vi "Get Test Limits Source File Name.vi"(8 "error in (no error)":errorcluster, 11 "Path":path) -> (0 "error out":errorcluster, 3 "Source File":string)   [LabVIEW 2025, in "File System.lvlib"]
uses:
  File System.lvlib
  <vilib>/Utility/file.llb/Read Delimited Spreadsheet (string).vi
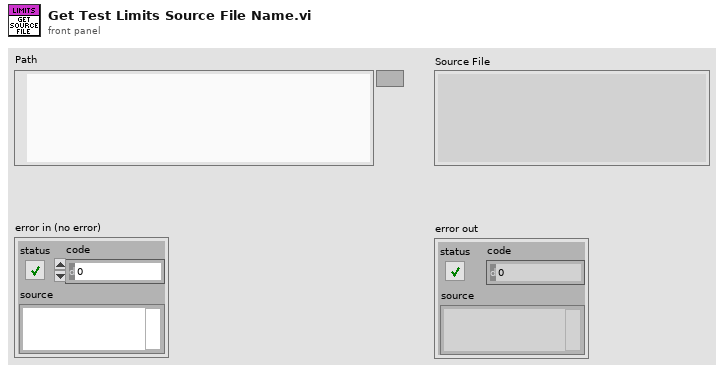
[diagram p1: front panel]
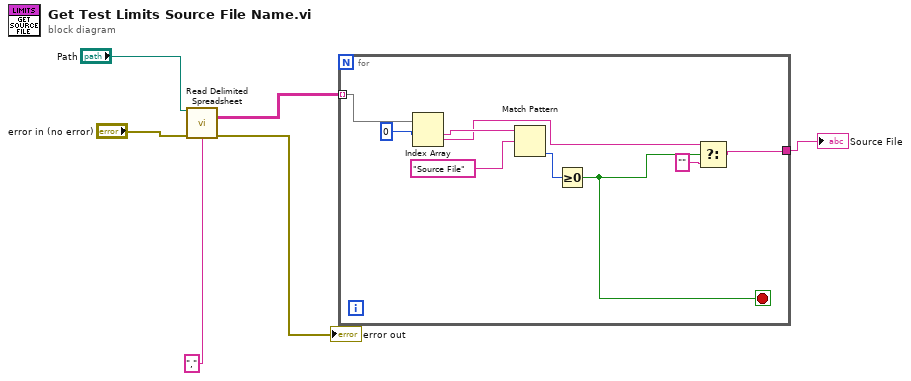
[diagram p0: block diagram]
diagram:
  n1 = call-poly <vilib>:"Read Delimited Spreadsheet.vi"("file path (dialog if empty)"="Path", "error in (no error)"="error in (no error)", "delimiter (\\t)"="," ("delimiter (\\t)")) -> ("all rows"=w2:string[][], "error out"=→"error out":errorcluster)  [unwired: 7 in, 4 out]
  n2 = for {
    tunnel: w2 -> [w15] mode=indexing
    tunnel: [w7] -> w1
    stop <- w10 stop-if-true
    n3 = Index Array(array=w15, index #1=0 ("index")) -> (element #1=w13:string, element #2=w9:string)  [unwired: 1 in]
    n4 = Match Pattern(string=w13, regular expression="Source File") -> (offset past match=w11:i32)  [unwired: 1 in, 3 out]
    n5 = Greater Or Equal To 0?(x=w11) -> (x >= 0?=w10:bool)
    n6 = Select(t=w9, s=w10, f="") -> (s? t:f=w7:string)
  }
  "Source File" <- w1
